vi "ExPhotometricsAsync2.vi"() -> ()   [LabVIEW 2010]
panel:
  in  "PMode":dbl(ring)=1.0 items=["n/a", "Normal", "FT", "Normal MPP", "FT MPP", "Alt Normal", "Alt FT", "Alt Normal MPP", "Alt FT MPP", "Interline"]
  in  "Shutter end state":u32(ring)=1 items=["N/A", "No Change (keep cc and shutter as is)", "Halt (No Cont Clears)", "Halt Close shutter (No cont. clears)", "Clear (turn on cont clears)", "Clear and close shutter (cc on, shutter closed)", "Open shutter (no cont clears)", "Clear and open shutter (cc on, shutter open)", ""]
  in  "Shutter State":u32(ring)=1 items=["N/A", "Shutter always closed.", "Shutter Normal (open for expos/close for readout)", "Shutter opened begin acquisition sequence", "Shutter open prior-trigger"]
  in  "Trigger Edge":u32(ring)=1 items=["N/A", "Positive (leading) edge", "Negative (falling) edge"]
  in  "Timing Mode":u32(ring)=1
  in  "Exposure":dbl min=0.0 step=0.001 format="%.3f"
  in  "stop":bool
  in  "Store":bool
  out "error out":errorcluster
  in  "error in (no error)":errorcluster
  # "ExPhotometricsAsync2:\nThis is a Full Frame Async example dessigned specificly for \nPhotometrics cameras. This should work with \nall camera systems. It requires a start for every frame \ncollected. Not all timing modes work for all cameras, also \nthe trigger edge only applies to Princeton Instrument \ncameras. Not all cameras have the ability to set the \ntemperature.\nPressing the stop button stops the example.\nThis example shows how to set PMode."
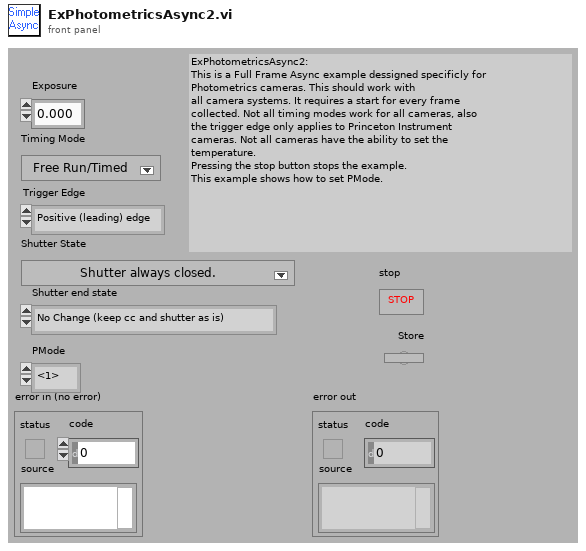
[diagram p1: front panel]
types:
  T1 = cluster{"Acquire mode \n3 is Async":i32, "Exposure":dbl, "Number of Images":i32, "Software Accums":i32}
  T2 = cluster{"Camera Handle":u32, "Pulser Handle":u32, "File Handle":u32, "Display Handle":u32, "Image Handle":u32}
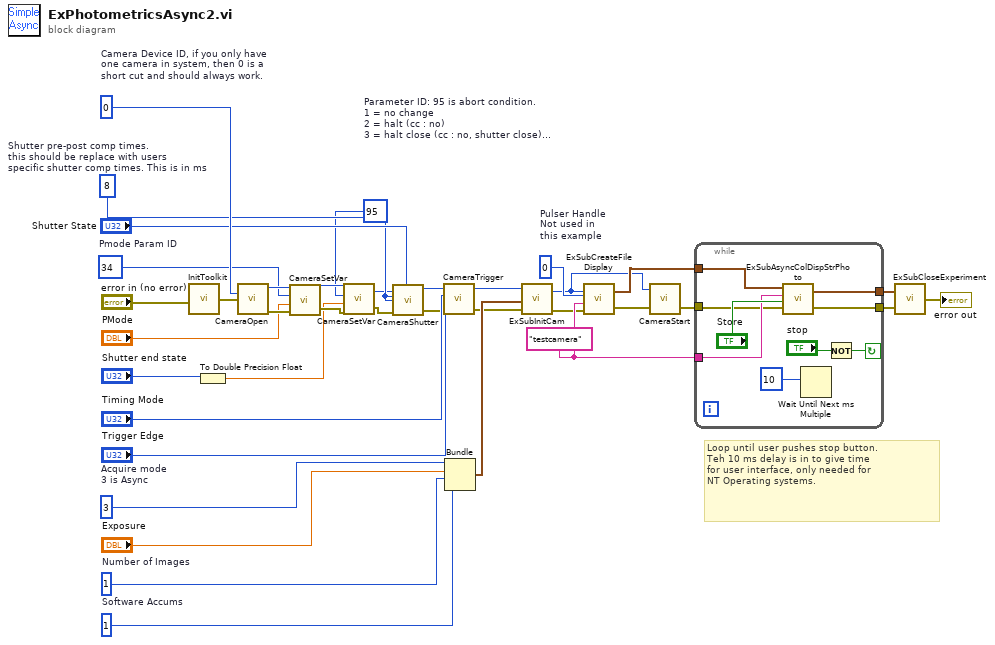
[diagram p0: block diagram]
diagram:
  w11 = 34  # Pmode Param ID
  w1 = 95  # Parameter ID: 95 is abort condition. 1 = no change 2 = halt (cc : no) 3 = halt close (cc : no, shutter close) 4 = clear (cc : yes) 5 = clear close (cc : yes, shutter close) 6 = open (cc : no, shutter open) 7 = clear open (cc : yes, shutter open)
  w17 = 8  # Shutter pre-post comp times. this should be replace with users  specific shutter comp times. This is in ms
  w23 = 0  # Camera Device ID, if you only have  one camera in system, then 0 is a  short cut and should always work.
  w30 = 0  # Pulser Handle Not used in  this example
  w35 = 1  # Number of Images
  w36 = 3  # Acquire mode  3 is Async
  w34 = 1  # Software Accums
  w37 = "testcamera"
  # "Loop until user pushes stop button.\nTeh 10 ms delay is in to give time \nfor user interface, only needed for \nNT Operating systems."
  n1 = call <userlib>:"InitToolkit.vi"("error in"="error in (no error)") -> ("error out"=w24:errorcluster)
  n2 = To Double Precision Float(number="Shutter end state") -> (double precision float=w6:dbl)
  n3 = call <userlib>:"CameraOpen.vi"("error in"=w24, "Camera Device ID"=w23) -> ("error out"=w14:errorcluster, "Camera Handle"=w13:u32)
  n4 = call <userlib>:"CameraSetVar.vi"("error in"=w14, "Value"="PMode", "Parameter ID"=w11, "Camera Handle"=w13) -> ("error out"=w8:errorcluster, "CameraHandle"=w7:u32)
  n5 = call <userlib>:"CameraSetVar.vi"("error in"=w8, "Value"=w6, "Parameter ID"=w1, "Camera Handle"=w7) -> ("error out"=w4:errorcluster, "CameraHandle"=w5:u32)
  n6 = call <userlib>:"CameraShutter.vi"("Camera Handle"=w5, "Shutter Comp Time: Pre Open"=w17, "Shutter Comp Time: Post Open"=w17, "error in"=w4, "Shutter State"="Shutter State") -> ("Camera Handle"=w3:u32, "error out"=w2:errorcluster)
  n7 = call <userlib>:"CameraTrigger.vi"("error in"=w2, "Trigger Edge"="Trigger Edge", "Timing Mode"="Timing Mode", "Camera Handle"=w3) -> ("error out"=w20:errorcluster, "Camera Handle"=w19:u32)
  n8 = Bundle("Acquire mode \n3 is Async"=w36, "Exposure"="Exposure", "Number of Images"=w35, "Software Accums"=w34) -> (w32:T1)  [unwired: 1 in]
  n9 = call "ExSubInitCam.vi"("error in (no error)"=w20, "Camera Information"=w32, "Camera Handle"=w19) -> ("error out"=w31:errorcluster, "Camera Handle"=w10:u32)
  n10 = call "ExSubCreateFileDisplay.vi"("error in (no error)"=w31, "File and Display Name"=w37, "Pulser Handle"=w30, "Camera Handle"=w10) -> ("error out"=w9:errorcluster, "Handles Out"=w15:T2)
  n11 = call <userlib>:"CameraStart.vi"("error in"=w9, "Camera Handle"=w10) -> ("error out"=w29:errorcluster)  [unwired: 1 out]
  n12 = while {
    tunnel: w15 -> [w44]
    tunnel: w29 -> [w42]
    tunnel: w37 -> [w43]
    tunnel: [w40] -> w27
    tunnel: [w41] -> w28
    stop <- w39 continue-if-true
    n13 = call "ExSubAsyncColDispStrPhoto.vi"("error in (no error)"=w42, "Store Data"="Store", "Display Title"=w43, "Handle Cluster"=w44) -> ("error out"=w40:errorcluster, "Handle Cluster Out"=w41:T2)
    n14 = Wait Until Next ms Multiple(millisecond multiple=10) -> ()  [unwired: 1 out]
    n15 = Not(x="stop") -> (.not. x?=w39:bool)
  }
  n16 = call "ExSubCloseExperiment.vi"("error in (no error)"=w27, "Handles In"=w28) -> ("error out"=→"error out":errorcluster)
